vi "Construct Category Menu.vi"(8 "error in (no error)":errorcluster, 10 "Categories":refnum<class "Category.lvclass">[](array[class]), 11 "Menu in":refnum<k9>) -> (0 "error out":errorcluster)   [LabVIEW 2018]
uses:
  classes/Category/Category.lvclass
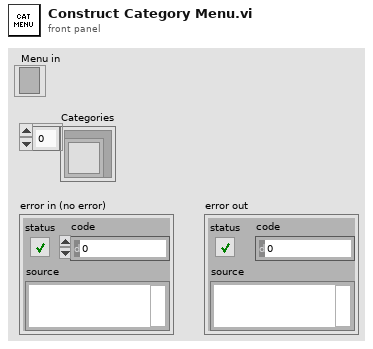
[diagram p1: front panel]
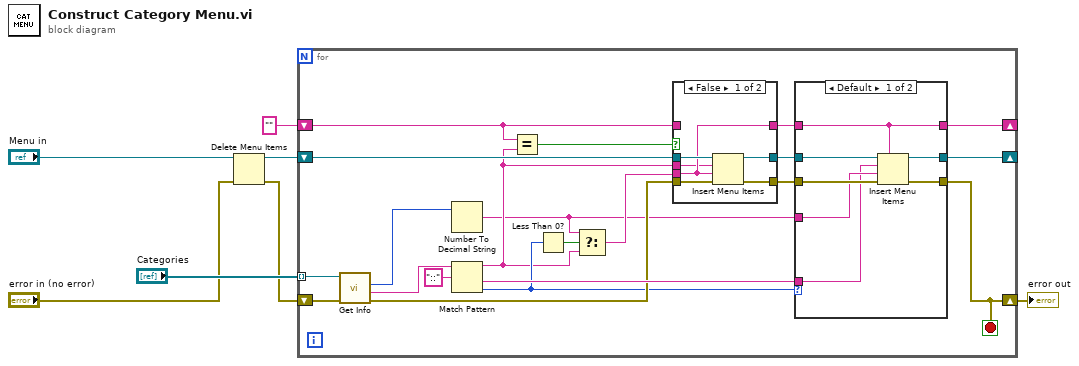
[diagram p0: block diagram]
diagram:
  n1 = Delete Menu Items(6:"error in (no error)", 9:"Menu in") -> (0:w6:errorcluster, 3:w4:refnum<k9>)  [unwired: 2 in]
  n2 = for {
    shift-right: [w26] -> w2
    shift-left: w6 -> [w19]
    shift-right: [w22] -> _
    shift-left: w4 -> [w27]
    shift-right: [w10] -> _
    shift-left: "" -> [w20]
    tunnel: "Categories" -> [w18] mode=indexing
    stop <- w26 stop-if-true
    n3 = call "Get Info.vi"("error in (no error)"=w19, "Category in"=w18) -> ("error out"=w17:errorcluster, "Name"=w16:string, "id"=w15:i32)  [unwired: 6 in, 1 out]
    n4 = Number To Decimal String(number=w15) -> (decimal integer string=w8:string)  [unwired: 1 in]
    n5 = Match Pattern(string=w16, regular expression="::") -> (before substring=w12:string, after substring=w24:string, offset past match=w14:i32)  [unwired: 1 in, 1 out]
    n6 = Equal?(x=w20, y=w12) -> (x = y?=w21:bool)
    n7 = Less Than 0?(x=w14) -> (x < 0?=w13:bool)
    n8 = Select(t=w8, s=w13, f=w12) -> (s? t:f=w9:string)
    n9 = case shown="False" w21 {
      tunnel: w27 -> [w34 w37]
      tunnel: w17 -> [w33 w36]
      tunnel: [w32 w36] -> w25
      tunnel: [w31 w37] -> w23
      tunnel: w12 -> [w29 _]
      tunnel: w20 -> [_ w35]
      tunnel: w9 -> [w30 _]
      tunnel: [w30 w35] -> w11
      frame False {
        n10 = Insert Menu Items(6:w33, 7:w30, 8:w29, 9:w34) -> (0:w32:errorcluster, 3:w31:refnum<k9>)  [unwired: 2 in, 1 out]
      }
      frame True {
      }
    }
    n11 = case shown="Default" w14 {
      tunnel: [w43 w47] -> w26
      tunnel: w25 -> [w44 w47]
      tunnel: w24 -> [w38 _]
      tunnel: w23 -> [w42 w46]
      tunnel: [w41 w46] -> w22
      tunnel: w11 -> [w40 w45]
      tunnel: [w40 w45] -> w10
      tunnel: w8 -> [w39 _]
      frame Default {
        n12 = Insert Menu Items(5:w40, 6:w44, 7:w39, 8:w38, 9:w42) -> (0:w43:errorcluster, 3:w41:refnum<k9>)  [unwired: 1 in, 1 out]
      }
      frame -1 {
      }
    }
  }
  "error out" <- w2
